vi "PV ActiveLine - Baudrate.vi"(7 "W/R":bool, 8 "Fehler (Eingang)":errorcluster, 9 "Baud Rate":u32(ring) items=["9600 (default)", "19200", "38400", "57600", "115200"], 11 "Referenz in":refnum<visa-resource-name>) -> (0 "Cluster (Ausgang)":errorcluster, 1 "Baud Rate out":u32(ring) items=["9600 (default)", "19200", "38400", "57600", "115200"], 2 "Read Status":u16(ring) items=["Read Failed", "Read Ok"], 3 "Referenz out":refnum<visa-resource-name>)   [LabVIEW 2013, in "PV ActiveLine.lvlib"]
doc: "BAU - Transmission Rate\n\nTransmit: BAU [,a]\nReceive: a\n\nTransmission rate, a =\n0 –> 9600 Baud (default)\n1 –> 19200 Baud\n2 –> 38400 Baud\n3 –> 57600 Baud\n4 –> 115200 Baud\n\nThe transmission rate of the RS485 (pv protocol) interface is 9600 baud and cannot be changed.\n\nAs soon as the new baud rate has been entered, the report signal is transmitted at the new transmission rate."
uses:
  <instrlib>/PV ActiveLine/PV ActiveLine.lvlib
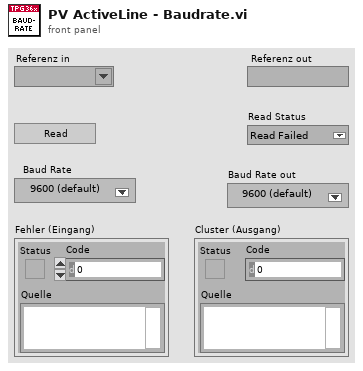
[diagram p1: front panel]
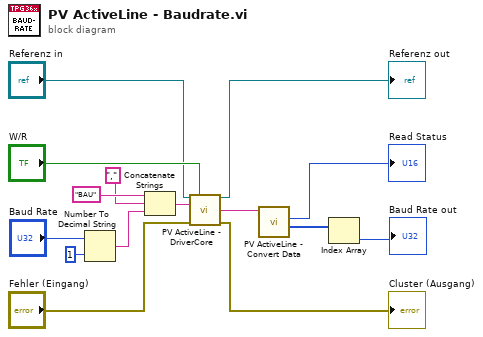
[diagram p0: block diagram]
diagram:
  n1 = Number To Decimal String(number="Baud Rate", width (-)=i16 1) -> (decimal integer string=w13:string)
  n2 = Concatenate Strings("BAU" ("Command"), "," ("Command"), w13) -> (w10:string)
  n3 = call <instrlib>:"PV ActiveLine - DriverCore.vi"("Referenz in"="Referenz in", "Write/Read"="W/R", "Command"=w10, "Fehler (Eingang)"="Fehler (Eingang)") -> ("Referenz out"=→"Referenz out":refnum<visa-resource-name>, "String Out"=w5:string, "Cluster (Ausgang)"=→"Cluster (Ausgang)":errorcluster)  [unwired: 9 in]
  n4 = call <instrlib>:"PV ActiveLine - Convert Data.vi"("String in"=w5) -> ("Integer Out"=w3:i32[], "Read Status"=→"Read Status":u16)  [unwired: 7 in, 2 out]
  n5 = Index Array(array=w3) -> (element=→"Baud Rate out":i32)  [unwired: 1 in]
